vi "Heat.vi"() -> ()   [LabVIEW 2014]
uses:
  Controls/Conveyor Belt Functions.ctl
panel:
  in  "Heat Position Sensor":tag[](array[tag])
  in  "Conv. Belt Pin":tag
  out "error out 2":errorcluster
  in  "error in (no error)":errorcluster
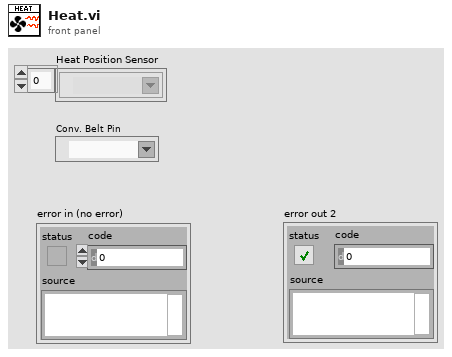
[diagram p1: front panel]
types:
  T1 = typedef "Conveyor Belt Functions.ctl" = enum16{"Move Forward", "Move Backward", "Stop"}
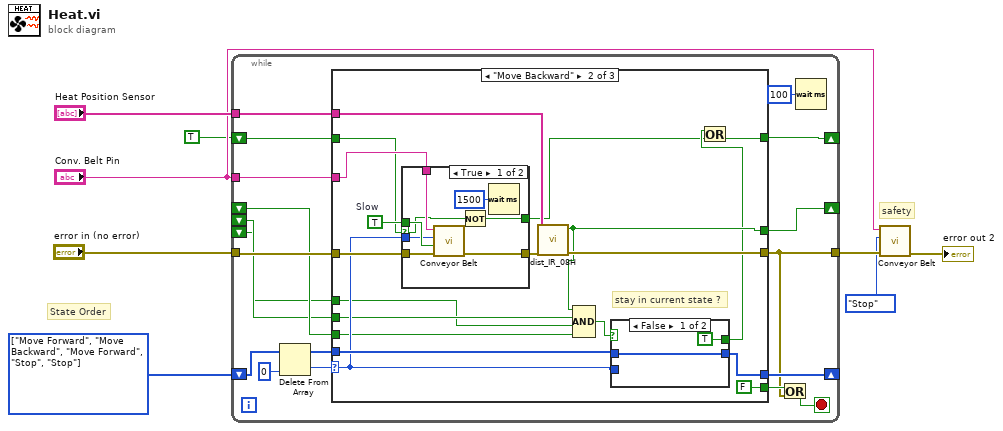
[diagram p0: block diagram]
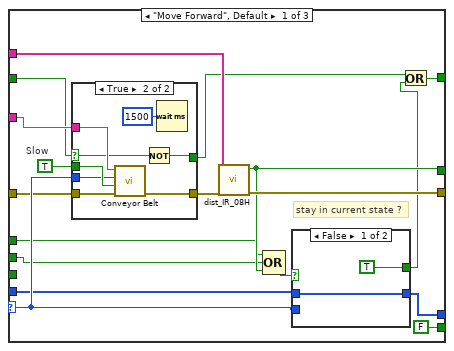
[diagram p2: hidden frame]
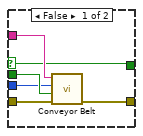
[diagram p3: hidden frame]
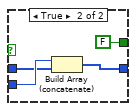
[diagram p4: hidden frame]
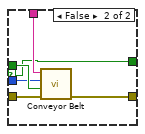
[diagram p5: hidden frame]
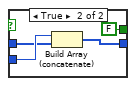
[diagram p6: hidden frame]
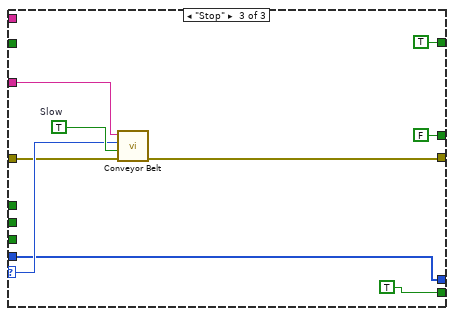
[diagram p7: hidden frame]
diagram:
  w8 = T1[] [enum."Move Forward", enum."Move Backward", enum."Move Forward", enum."Stop", enum."Stop"] items=["Move Forward", "Move Backward", "Stop"]
  # "safety"
  # "State Order"
  n1 = while {
    shift-right: [w22] -> _
    shift-left: w8 -> [w26]
    tunnel: "error in (no error)" -> [w21]
    tunnel: [w17] -> w5
    tunnel: "Conv. Belt Pin" -> [w20]
    tunnel: "Heat Position Sensor" -> [w19]
    shift-right: [w14] -> _
    shift-left: _ -> [w13]
    shift-left: _ -> [w12]
    shift-left: _ -> [w11]
    shift-right: [w10] -> _
    shift-left: TRUE -> [w9]
    stop <- w16 stop-if-true
    n2 = Delete From Array(array=w26, index=0) -> (deleted portion=w23:T1, array with subset deleted=w24:T1[])  [unwired: 1 in]
    n3 = case shown="\"Move Backward\"" w23 {
      selector: w23 -> [w39 w75 w110]
      tunnel: w24 -> [w38 w83 w107]
      tunnel: [w36 w82 w107] -> w22
      tunnel: w21 -> [w37 w80 w109]
      tunnel: [w42 w79 w108] -> w17
      tunnel: w20 -> [w40 w77 w111]
      tunnel: w19 -> [w41 w76 _]
      tunnel: [FALSE ("Quit") FALSE ("Quit") TRUE] -> w18
      tunnel: [w33 w73 FALSE ("sensor signal (A/DIO0 (Pin 11))")] -> w14
      tunnel: w13 -> [_ w69 _]
      tunnel: w12 -> [w32 w71 _]
      tunnel: w11 -> [w31 w70 _]
      tunnel: w9 -> [w29 w68 _]
      tunnel: [w30 w67 TRUE] -> w10
      frame "Move Forward", Default {
        w44 = TRUE  # Slow
        # "stay in current state ?"
        n4 = case shown="True" w29 {
          selector: w29 -> [w45 w52]
          tunnel: w44 -> [w50 w58]
          tunnel: [w49 w57] -> w43
          tunnel: w40 -> [w48 w56]
          tunnel: w39 -> [w47 w55]
          tunnel: w37 -> [w46 w54]
          tunnel: [w45 w51] -> w27
          frame False {
            n5 = call "Conveyor Belt.vi"("error in (no error)"=w46, "Slow"=w50, "Function"=w47, "Conv. Belt Pin"=w48) -> ("error out"=w49:errorcluster)  [unwired: 7 in]
          }
          frame True {
            n6 = call "Conveyor Belt.vi"("error in (no error)"=w54, "Slow"=w58, "Function"=w55, "Conv. Belt Pin"=w56) -> ("error out"=w57:errorcluster)  [unwired: 7 in]
            n7 = Not(x=w52) -> (.not. x?=w51:bool)
            n8 = Wait (ms)(milliseconds to wait=u32 1500) -> ()  [unwired: 1 out]
          }
        }
        n9 = call "dist_IR_08H.vi"("error in (no error) 2"=w43, "Channel Names"=w41) -> ("error out 2"=w42:errorcluster, "sensor signal (A/DIO0 (Pin 11))"=w33:bool)  [unwired: 8 in]
        n10 = Compound Arithmetic op=OR(w31, w32, w33) -> (w34:bool)
        n11 = case shown="False" w34 {
          tunnel: [w60 w64] -> w36
          tunnel: w39 -> [_ w63]
          tunnel: w38 -> [w60 w62]
          tunnel: [TRUE FALSE] -> w28
          frame False {
          }
          frame True {
            n12 = Build Array (concatenate) ("Array erstellen")(w63, w62) -> (w64:T1[])
          }
        }
        n13 = Or(x=w27, y=w28) -> (x .or. y?=w30:bool)
      }
      frame "Move Backward" {
        w78 = TRUE  # Slow
        # "stay in current state ?"
        n14 = case shown="True" w68 {
          selector: w68 -> [w85 w92]
          tunnel: [w91 w97] -> w81
          tunnel: w80 -> [w90 w96]
          tunnel: w78 -> [w89 w95]
          tunnel: w77 -> [w88 w94]
          tunnel: w75 -> [w87 w93]
          tunnel: [w84 w92] -> w65
          frame True {
            n15 = call "Conveyor Belt.vi"("error in (no error)"=w90, "Slow"=w89, "Function"=w87, "Conv. Belt Pin"=w88) -> ("error out"=w91:errorcluster)  [unwired: 7 in]
            n16 = Not(x=w85) -> (.not. x?=w84:bool)
            n17 = Wait (ms)(milliseconds to wait=u32 1500) -> ()  [unwired: 1 out]
          }
          frame False {
            n18 = call "Conveyor Belt.vi"("error in (no error)"=w96, "Slow"=w95, "Function"=w93, "Conv. Belt Pin"=w94) -> ("error out"=w97:errorcluster)  [unwired: 7 in]
          }
        }
        n19 = call "dist_IR_08H.vi"("error in (no error) 2"=w81, "Channel Names"=w76) -> ("error out 2"=w79:errorcluster, "sensor signal (A/DIO0 (Pin 11))"=w73:bool)  [unwired: 8 in]
        n20 = Compound Arithmetic op=AND(w73, w71, w70, w69) -> (w72:bool)
        n21 = case shown="False" w72 {
          tunnel: [w99 w103] -> w82
          tunnel: w75 -> [_ w102]
          tunnel: w83 -> [w99 w101]
          tunnel: [TRUE FALSE] -> w66
          frame False {
          }
          frame True {
            n22 = Build Array (concatenate) ("Array erstellen")(w102, w101) -> (w103:T1[])
          }
        }
        n23 = Or(x=w66, y=w65) -> (x .or. y?=w67:bool)
      }
      frame "Stop" {
        w112 = TRUE  # Slow
        n24 = call "Conveyor Belt.vi"("error in (no error)"=w109, "Slow"=w112, "Function"=w110, "Conv. Belt Pin"=w111) -> ("error out"=w108:errorcluster)  [unwired: 7 in]
      }
    }
    n25 = Or(x=w18, y=w17) -> (x .or. y?=w16:bool)
    n26 = Wait (ms)(milliseconds to wait=u32 100) -> ()  [unwired: 1 out]
  }
  n27 = call "Conveyor Belt.vi"("error in (no error)"=w5, "Function"=Conveyor_Belt_Functions."Stop", "Conv. Belt Pin"="Conv. Belt Pin") -> ("error out"=→"error out 2":errorcluster)  [unwired: 8 in]
